vi "DCIR_HPPC_Create.vi"(0 "reference in":refnum<class "DCIR_HPPC.lvclass">, 5 "HPPC Parameters":T1={"HPPC Mode"=1, "Pulse Duration (S)"=500.0, "Charge Current (A)"=1000.0, "Rest Duration (S)"=2.0, "Discharge Current (A)"=10.0, "Temperature (C)"=25.0, "Nominal Capacity (Ah)"=10.0, "Initial SoC (%)"=650.0, "Final SoC (%)"=50.0, "SoC Interval (%)"=10.0, "SoC Step Current (A)"=10.0, "SoC Step Relax (S)"=10.0} {"HPPC Mode" items=["One Shot (DCIR)", "Discharge Only", "Full Cycle"]; "Nominal Capacity (Ah)" min=0.0 max=100.0; "Final SoC (%)" min=0.0 max=100.0; "SoC Interval (%)" min=0.0 max=100.0; "Initial SoC (%)" min=0.0 max=100.0}, 7 "Logger":refnum<class "Logger.lvclass">, 9 "Power Module":refnum<class "PowerModuleInterface.lvclass">, 11 "Error In":errorcluster) -> (4 "reference out":refnum<class "DCIR_HPPC.lvclass">, 6 "ProcessViRef":refnum<vi>, 15 "Error Out":errorcluster)   [LabVIEW 2023, in "DCIR_HPPC.lvclass"]
uses:
  DCIR_HPPC.lvclass
  Logger_class/Logger.lvclass
  builds/PowerModuleInterface/PowerModuleInterface.lvlibp/Classes/PowerModule_interface/PowerModuleInterface.lvclass
  HPPC Parameters.ctl
  HPPC Mode.ctl
  DCIR_HPPC.lvclass/DCIR_HPPC.ctl
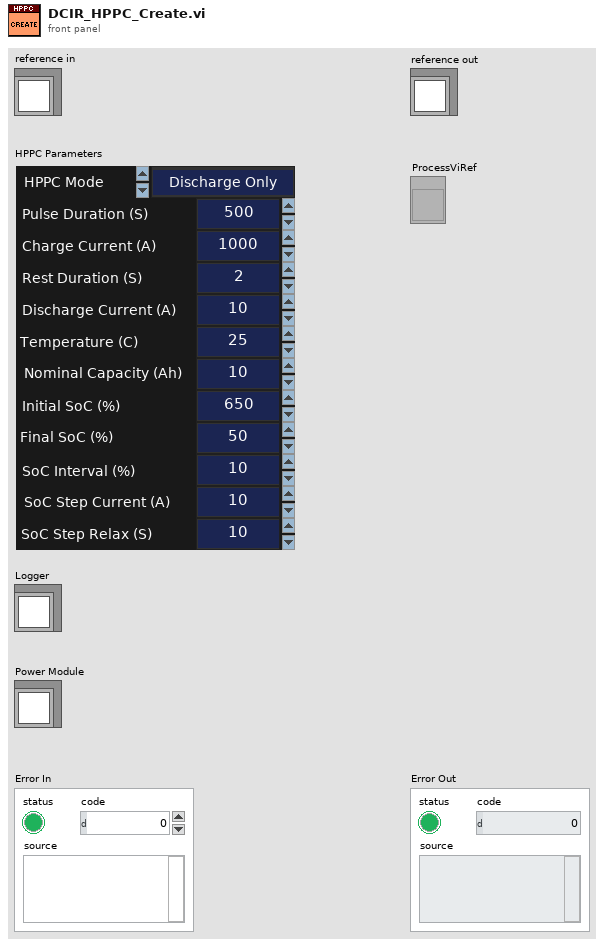
[diagram p1: front panel]
types:
  T1 = typedef "DCIR_HPPC.lvclass/HPPC Parameters.ctl" = cluster{"HPPC Mode":T2, "Pulse Duration (S)":dbl, "Charge Current (A)":dbl, "Rest Duration (S)":dbl, "Discharge Current (A)":dbl, "Temperature (C)":dbl, "Nominal Capacity (Ah)":dbl, "Initial SoC (%)":dbl, "Final SoC (%)":dbl, "SoC Interval (%)":dbl, "SoC Step Current (A)":dbl, "SoC Step Relax (S)":dbl}
  T2 = typedef "DCIR_HPPC.lvclass/HPPC Mode.ctl" = u16
  T3 = typedef "DCIR_HPPC.lvclass/ObjectAttributes.ctl" = cluster{"HPPC Parameters":T1, "Logger":refnum<class "Logger.lvclass">, "Power Module":refnum<class "PowerModuleInterface.lvclass">}
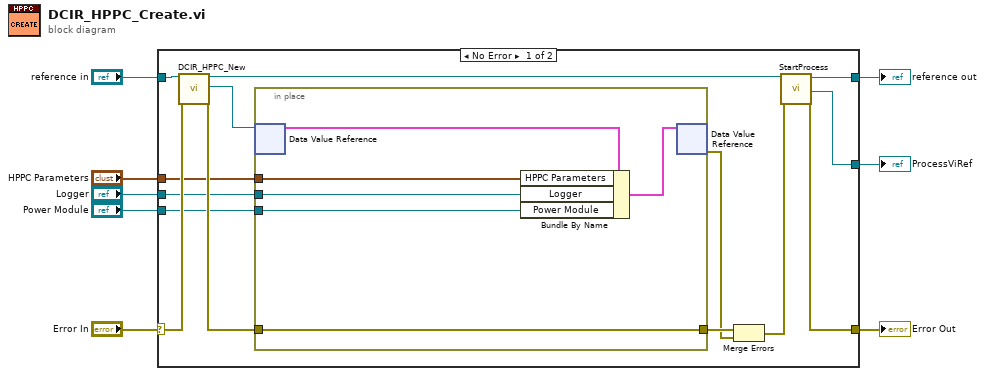
[diagram p0: block diagram]
diagram:
  n1 = case shown="No Error" "Error In" {
    selector: "Error In" -> [w21 w30]
    tunnel: [w15 w30] -> w7
    tunnel: "reference in" -> [w22 w29]
    tunnel: [w17 w29] -> w5
    tunnel: [w14 _] -> w4
    tunnel: "HPPC Parameters" -> [w13 _]
    tunnel: "Logger" -> [w10 _]
    tunnel: "Power Module" -> [w9 _]
    frame No Error {
      n2 = call "DCIR_HPPC_New.vi"("reference in"=w22, "Error In"=w21) -> ("reference out"=w18:refnum<class "DCIR_HPPC.lvclass">, "DVRRefOut"=w12:refnum<data-value>, "Error Out"=w20:errorcluster)  [unwired: 14 in, 1 out]
      n3 = in-place {
        in-place-border: w20 -> [w28]
        in-place-border: [w28] -> w19
        in-place-border: w13 -> [w23]
        in-place-border: w10 -> [w25]
        in-place-border: w9 -> [w24]
        n4 = in-place-dvr #1(w12) -> (w27:T3)  [unwired: 1 out]
        n5 = Bundle By Name(cluster=w27, "HPPC Parameters"=w23, "Logger"=w25, "Power Module"=w24) -> (w26:T3)
        n6 = in-place-dvr #1(w26) -> (w11:errorcluster)  [unwired: 1 out]
      }
      n7 = Merge Errors(w19, w11) -> (w16:errorcluster)
      n8 = call "StartProcess.vi"("reference in"=w18, "Error In"=w16) -> ("reference out"=w17:refnum<class "DCIR_HPPC.lvclass">, "ProcessViRef"=w14:refnum<vi>, "Error Out"=w15:errorcluster)  [unwired: 13 in, 2 out]
    }
    frame Error {
      # "VI-TechBaseTemplate_Simple_6x8x6"
    }
  }
  "Error Out" <- w7
  "reference out" <- w5
  "ProcessViRef" <- w4
